vi "delete element from control.vi"(8 "error in":errorcluster, 10 "control label":string, 11 "VI in":refnum<vi>) -> (0 "error out":errorcluster)   [LabVIEW 2013, in "FixedChannelTBModuleDecideFeatures.lvclass"]
uses:
  FixedChannelTBModuleDecideFeatures.lvclass
  <vilib>/Utility/traverseref.llb/TRef TravTarget.ctl
  <vilib>/Utility/traverseref.llb/VI Scripting - Traverse.lvlib
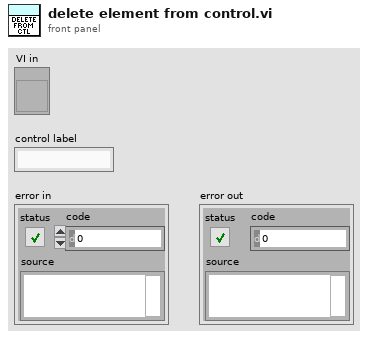
[diagram p1: front panel]
types:
  T1 = typedef "TRef TravTarget.ctl" = enum16{"FP", "BD", "Other"}
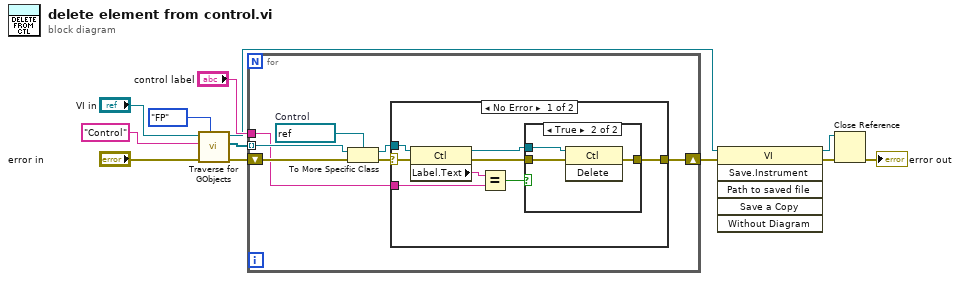
[diagram p0: block diagram]
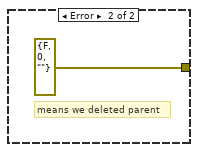
[diagram p3: hidden frame]
diagram:
  n1 = call <vilib>:"Traverse for GObjects.vi"("Traverse Target"=TRef_TravTarget."FP", "error in (no error)"="error in", "Class Name"="Control", "VI Refnum"="VI in") -> ("error out"=w8:errorcluster, "References"=w7:refnum<vi>[], "dup VI Refnum"=w4:refnum<vi>)  [unwired: 4 in, 1 out]
  n2 = for {
    tunnel: w7 -> [w18] mode=indexing
    tunnel: "control label" -> [w15]
    shift-right: [w14] -> w5
    shift-left: w8 -> [w19]
    w17 = refnum<vi> refnum  # Control
    n3 = To More Specific Class(target class=w17, reference=w18, error in=w19) -> (specific class reference=w16:refnum<vi>, error out=w13:errorcluster)
    n4 = case shown="No Error" w13 {
      selector: w13 -> [w20 _]
      tunnel: w16 -> [w27 _]
      tunnel: w15 -> [w25 _]
      tunnel: [w21 errorcluster {"status"=FALSE, "code"=0, "source"=""} ("error out")] -> w14
      frame No Error {
        n5 = property class="Ctl"(reference=w27, error in=w20) -> (reference out=w22:refnum<vi>, error out=w23:errorcluster, "Label.Text"=w26:string)
        n6 = Equal?(x=w26, y=w25) -> (x = y?=w24:bool)
        n7 = case shown="True" w24 {
          tunnel: w23 -> [w28 w31]
          tunnel: w22 -> [_ w30]
          tunnel: [w28 w29] -> w21
          frame False {
          }
          frame True {
            n8 = invoke class="Ctl" method="Delete"(reference=w30, error in=w31) -> (error out=w29:errorcluster)  [unwired: 1 in, 2 out]
          }
        }
      }
      frame Error {
        # "means we deleted parent"
      }
    }
  }
  n9 = invoke class="VI" method="Save.Instrument"(reference=w4, error in=w5) -> (reference out=w2:refnum<vi>, error out=w3:errorcluster)  [unwired: 4 in, 4 out]
  n10 = Close Reference(reference=w2, error in (no error)=w3) -> (error out=→"error out":errorcluster)
